vi "Init.vi"(8 "error in (no error)":errorcluster, 11 "CFG Base in":refnum<class "CFG Base.lvclass">) -> (0 "error out":errorcluster, 3 "CFG Base out":refnum<class "CFG Base.lvclass">)   [LabVIEW 2023, in "HAL GOOP4.lvlib" / "CFG Base.lvclass"]
uses:
  CFG Base.lvclass
  CFG Base.lvclass/CFG Base.ctl
  <vilib>/ErrorRing/Error Ring.xnode
  <vilib>/Utility/error.llb/Error Cluster From Error Code.vi
  D:/git/HAL/HAL GOOP4/Configuration/Configuration JSON/Configuration JSON Base/CFG JSON.lvclass
  D:/git/HAL/HAL GOOP4/Interfaces/IConfigure/IConfigure.lvclass
  D:/git/HAL/HAL GOOP4/Configuration/Configuration Base/CFG Base.lvclass
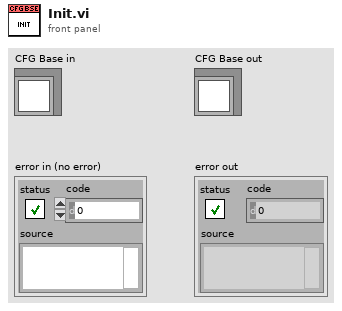
[diagram p1: front panel]
types:
  T1 = typedef "Semaphore RefNum" = refnum<k1>
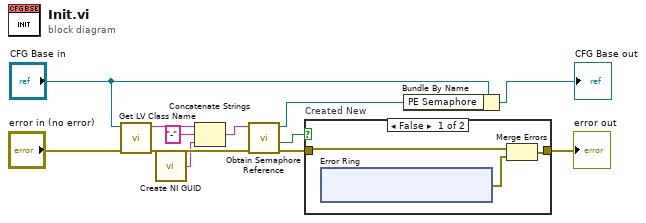
[diagram p0: block diagram]
diagram:
  n1 = call <vilib>:"Get LV Class Name.vi"("error in (no error)"="error in (no error)", "object"="CFG Base in") -> ("error out"=w11:errorcluster, "class name"=w10:string)  [unwired: 8 in]
  n2 = call <vilib>:"Create NI GUID.vi"() -> ("NI GUID"=w8:string)
  n3 = Concatenate Strings(w10, "-" ("string"), w8) -> (w7:string)
  n4 = call <vilib>:"Obtain Semaphore Reference.vi"("error in (no error)"=w11, "name (unnamed)"=w7) -> ("error out"=w6:errorcluster, "created new"=w5:bool, "semaphore"=w1:T1)  [unwired: 3 in]
  n5 = case "Created New" shown="False" w5 {
    tunnel: w6 -> [w13 w21]
    tunnel: [w15 w21] -> w4
    frame False {
      n6 = xnode "Error Ring"() -> ("error out"=w14:errorcluster)
      n7 = Merge Errors(w13, w14) -> (w15:errorcluster)
    }
    frame True {
    }
  }
  "error out" <- w4
  n8 = Bundle By Name(cluster="CFG Base in", "PE Semaphore"=w1) -> (→"CFG Base out":refnum<class "CFG Base.lvclass">)
